vi "Get_Tree.vi"(8 "error in (no error)":errorcluster, 11 "IB_Tree in":refnum<class "IB_Tree.lvclass">) -> (0 "error out":errorcluster, 2 "ctl":refnum<vi>, 3 "IB_Tree out":refnum<class "IB_Tree.lvclass">)   [LabVIEW 2020, in "IB_Tree.lvclass"]
uses:
  <vilib>/AppBuilder/IB_Classes/Tree/IB_Tree.lvclass
  <vilib>/AppBuilder/IB_Classes/Tree/IB_Tree.lvclass/IB_Tree.ctl
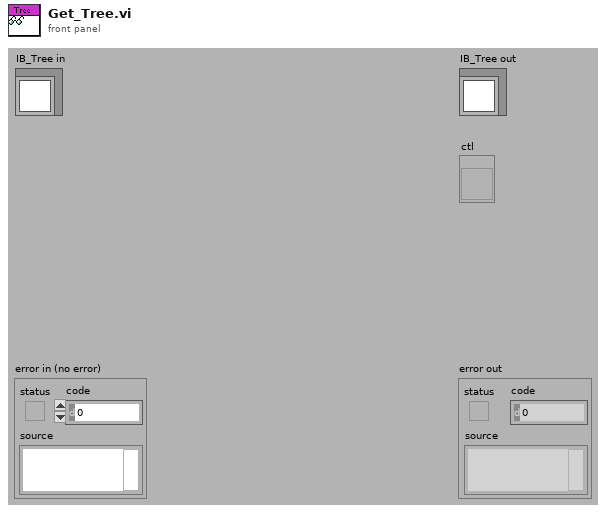
[diagram p1: front panel]
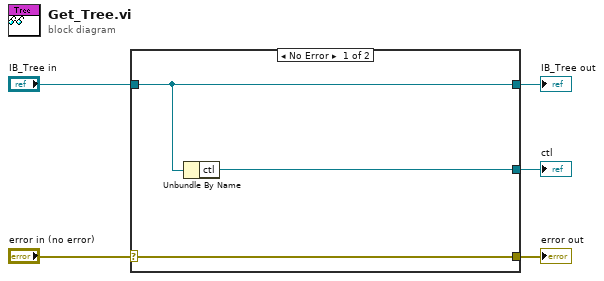
[diagram p0: block diagram]
diagram:
  n1 = case shown="No Error" "error in (no error)" {
    selector: "error in (no error)" -> [w8 w9]
    tunnel: [w8 w9] -> w4
    tunnel: [w7 w10] -> w2
    tunnel: "IB_Tree in" -> [w7 w10]
    tunnel: [w6 _] -> w1
    frame No Error {
      n2 = Unbundle By Name(w7) -> ("ctl"=w6:refnum<vi>)
    }
    frame Error {
    }
  }
  "error out" <- w4
  "IB_Tree out" <- w2
  "ctl" <- w1
